vi "Command_CRC.vi"(8 "error in (no error)":errorcluster caption="错误输入（无错误）", 10 "In":string) -> (0 "error out":errorcluster caption="错误输出", 2 "Out":string)   [LabVIEW 2015]
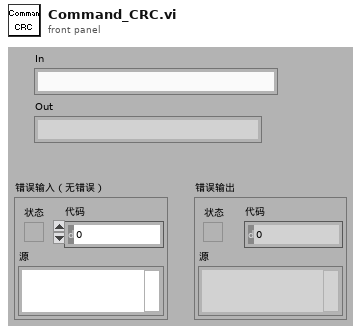
[diagram p1: front panel]
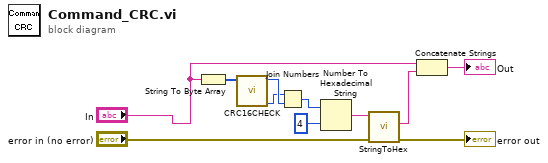
[diagram p0: block diagram]
diagram:
  n1 = String To Byte Array(string="In") -> (unsigned byte array=w6:u8[])
  n2 = call "CRC16CHECK.vi"("buf"=w6) -> ("CRCLo"=w3:u8, "CRCHi"=w4:u8)  [unwired: 9 out]
  n3 = Join Numbers(hi=w3, lo=w4) -> ((hi.lo)=w7:u16)
  n4 = Number To Hexadecimal String(1:i16 4 ("宽度(-)"), 2:w7) -> (0:w9:string)
  n5 = call "StringToHex.vi"("error in (no error)"="error in (no error)", "String_Hex"=w9) -> ("error out"=→"error out":errorcluster, "Hex"=w10:string)  [unwired: 8 out]
  n6 = Concatenate Strings("In", w10) -> (→"Out":string)
